vi "Write U32 value.vi"(8 "error in":errorcluster, 9 "value":u32, 10 "FPGA Setting":T2, 11 "FPGA ref":T1) -> (0 "error out":errorcluster, 3 "FPGA ref out":T1)   [LabVIEW 2013]
uses:
  FPGA/fpga_settings.ctl
  Scope/controls/settingsFPGAref.ctl
  <vilib>/rvi/interface/common/niFpgaWaitOnOcc.vi
  <vilib>/Utility/error.llb/Error Cluster From Error Code.vi
  <vilib>/rvi/errors/niLvFpgaAdjustHostInterfaceError.vi
  <vilib>/rvi/interface/nirviMethod/nirviMethod.xnode
  <vilib>/FPGAPlugInAG/Dynamic/niLvFpga_WriteFifo_Dynamic.vi
  <vilib>/rvi/errors/niLvFpgaMergeErrorWithErrorCode.vi
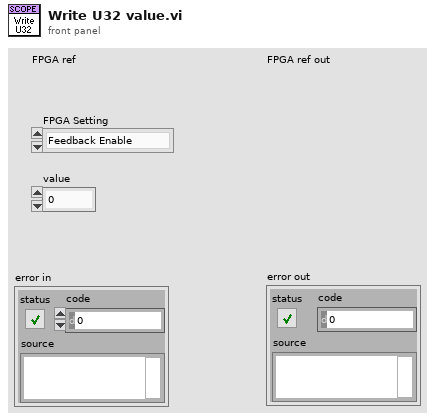
[diagram p1: front panel]
types:
  T1 = typedef "settingsFPGAref.ctl" = refnum<k20>
  T2 = typedef "fpga_settings.ctl" = enum16{"Feedback Enable", "New FIR coeffs", "FIR shift", "Enable filter", "Set Downsample", "Downsample", "CIC Gain", "Record length", "Trigger samples", "Quiet time", "a_am", "b_am", "Use fixed delay", "fixed sin_fi", "fixed cos_fi", "Ki*Tau", "Kp", "Kd_Tau", "Fi_start", "Fi_delta", "DC_offs 0", "DC_offs 1", "DC_offs 2", "DC_offs 3", "Ki*Tau am", "Kp am", "Kd_Tau am", "Feedback AM", "Trigger delay", "Feedback delay", "Setpoint enable", "Beam enable", "Samples to acquire", "Cavity Enable"}
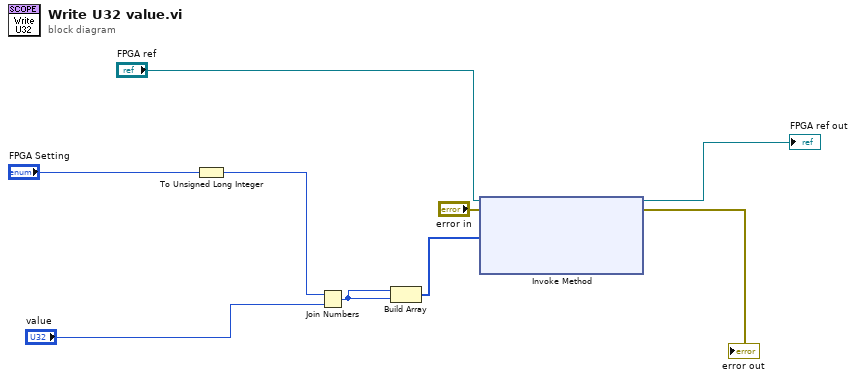
[diagram p0: block diagram]
diagram:
  n1 = To Unsigned Long Integer(number="FPGA Setting") -> (unsigned 32bit integer=w5:u32)
  n2 = Join Numbers(hi=w5, lo="value") -> ((hi.lo)=w4:u64)
  n3 = Build Array(w4, w4) -> (w6:u64[])
  n4 = xnode "Invoke Method"("FPGA VI Reference In"="FPGA ref", "error in"="error in", "Data"=w6) -> ("FPGA VI Reference Out"=→"FPGA ref out":T1, "error out"=→"error out":errorcluster)  [unwired: 1 in, 1 out]
